vi "Export Scenario List.vi"(8 "error in (no error)":errorcluster, 11 "Node Ptr":u64 format="%.0x") -> (0 "error out":errorcluster)   [LabVIEW 2023, in "Vires VTD System Explorer.lvlib"]
uses:
  Vires VTD System Explorer.lvlib
  Shared/Constants.vi
  <vilib>/NI VeriStand/Custom Device API/Get Item Property (String Array).vi
  <vilib>/Utility/file.llb/Write Delimited Spreadsheet (string).vi
  <vilib>/NI VeriStand/Custom Device API/Custom Device API.lvlib
  Shared/Vires VTD Shared.lvlib
  <vilib>/NI VeriStand/Custom Device Tools/Custom Device Utility Library/Custom Device Utility Library.lvlib
panel:
  in  "Tag":string
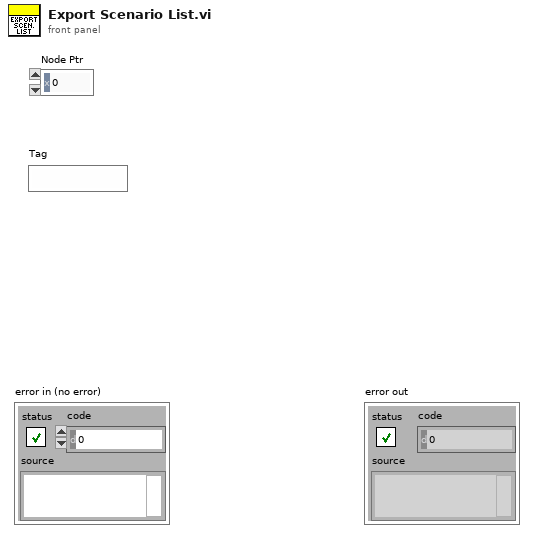
[diagram p1: front panel]
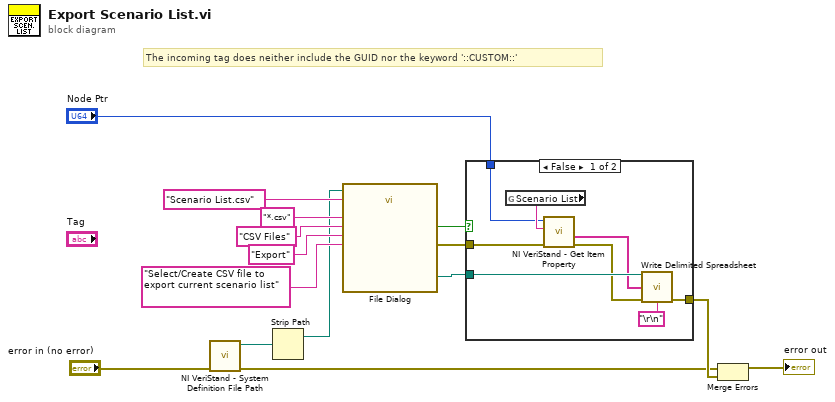
[diagram p0: block diagram]
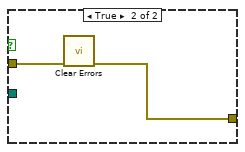
[diagram p2: hidden frame]
diagram:
  # "The incoming tag does neither include the GUID nor the keyword '::CUSTOM::'"
  n1 = call <vilib>:"NI VeriStand - System Definition File Path.vi"("error in (no error)"="error in (no error)") -> ("error out"=w2:errorcluster, "SDF path"=w4:path)  [unwired: 9 in]
  n2 = Strip Path(path=w4) -> (stripped path=w1:path)  [unwired: 1 out]
  n3 = call "File Dialog"("start path"=w1, "prompt"="Select/Create CSV file to export current scenario list", "button label"="Export", "default name"="Scenario List.csv", "pattern (all files)"="*.csv", "pattern label"="CSV Files") -> ("selected path"=w9:path, "cancelled"=w10:bool, "error out"=w8:errorcluster)  [unwired: 6 in, 1 out]
  n4 = case shown="False" w10 {
    tunnel: w9 -> [w23 _]
    tunnel: w8 -> [w17 w25]
    tunnel: [w21 w24] -> w7
    tunnel: "Node Ptr" -> [w19 _]
    frame False {
      n5 = global read "Constants.vi" "Scenario List"() -> (w20:string)
      n6 = call-poly <vilib>:"NI VeriStand - Get Item Property.vi"("error in (no error)"=w17, "Property Name"=w20, "Item Ref in"=w19) -> ("error out"=w16:errorcluster, "Value"=w18:string[])  [unwired: 5 in, 2 out]
      n7 = call-poly <vilib>:"Write Delimited Spreadsheet.vi"("file path (dialog if empty)"=w23, "1D data"=w18, "error in (no error)"=w16, "delimiter (\\t)"="\r\n") -> ("error out"=w21:errorcluster)  [unwired: 10 in, 1 out]
    }
    frame True {
      n8 = call <vilib>:"Clear Errors.vi"("error in (no error)"=w25) -> ("error out"=w24:errorcluster)  [unwired: 5 in, 1 out]
    }
  }
  n9 = Merge Errors(w2, w7) -> (→"error out":errorcluster)
